vi "SFOAE-Compute Stim Spectra.vi"(0 "DataProc In":T1, 1 "MagSpect In":cluster{"Array":dbl[], "Array":dbl[]}[](array[cluster]), 11 "error in (no error)":errorcluster, 13 "Smoothing":cluster{"Length":i32, "Iterations":i32}={"Length"=1, "Iterations"=1}) -> (3 "MagSpect":cluster{"Array":dbl[], "Array":dbl[]}[](array[cluster]), 4 "DataProc Out":T1, 15 "error out":errorcluster)   [LabVIEW 2020]
uses:
  Typedefs/SFOAE-Data Processing.ctl
  <vilib>/Analysis/baseanly.llb/Mean (DBL).vi
  epl-vi-lib/Utility VIs/Math VIs/FFT x(t) to dB,Degrees (1D).vi
  epl-vi-lib/Utility VIs/Math VIs/Linear to dB (array).vi
  <vilib>/Analysis/NI_AALBase.lvlib
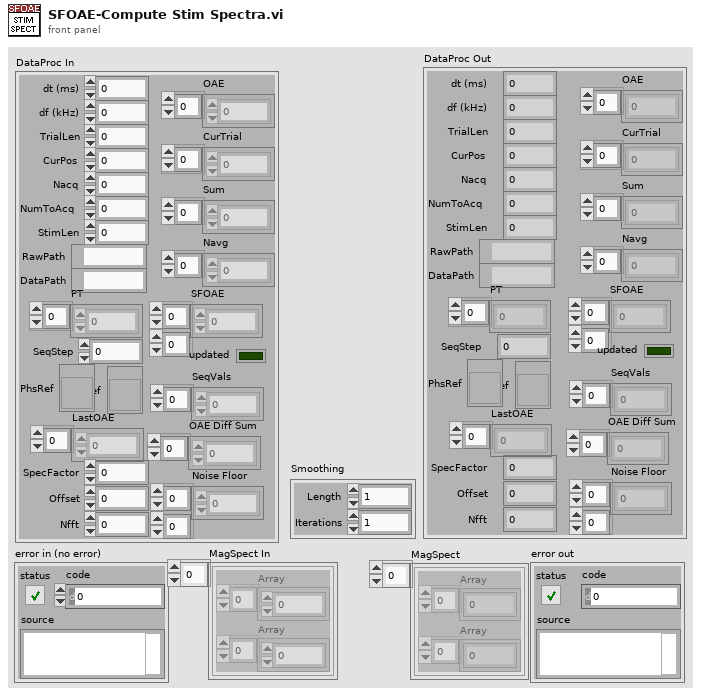
[diagram p1: front panel]
types:
  T1 = typedef "SFOAE-Data Processing.ctl" = cluster{"dt (ms)":dbl, "TrialLen":i32, "PT":cdb[], "CurPos":i32, "Sum":dbl[], "Navg":dbl[], "Nacq":i32, "RawPath":path, "DataPath":path, "NumToAcq":i32, "OAE":dbl[], "CurTrial":dbl[], "StimLen":i32, "SFOAE":cdb[][], "SeqStep":i32, "updated":bool, "SeqVals":dbl[], "df (kHz)":dbl, "MagRef":refnum<vi>, "LastOAE":dbl[], "OAE Diff Sum":dbl[], "Noise Floor":cdb[][], "SpecFactor":dbl, "Offset":i32, "Nfft":i32, "PhsRef":refnum<vi>}
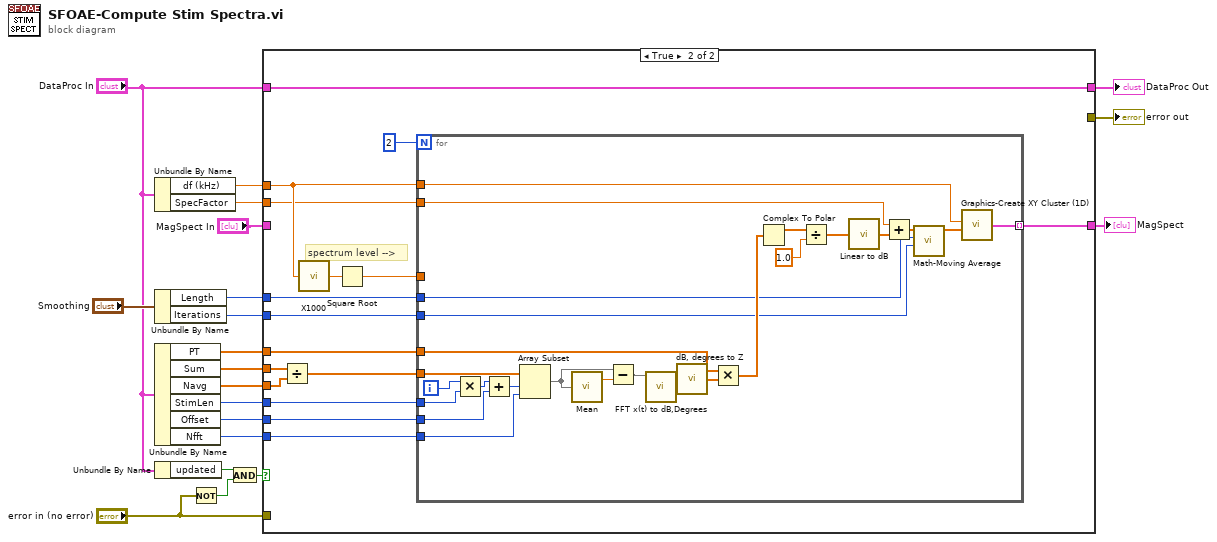
[diagram p0: block diagram]
diagram:
  n1 = Unbundle By Name("DataProc In") -> ("df (kHz)"=w13:dbl, "SpecFactor"=w8:dbl)
  n2 = Unbundle By Name("Smoothing") -> ("Length"=w11:i32, "Iterations"=w10:i32)
  n3 = Unbundle By Name("DataProc In") -> ("PT"=w6:cdb[], "Sum"=w14:dbl[], "Navg"=w7:dbl[], "StimLen"=w5:i32, "Offset"=w2:i32, "Nfft"=w1:i32)
  n4 = Unbundle By Name("DataProc In") -> ("updated"=w18:bool)
  n5 = Not(x="error in (no error)") -> (.not. x?=w17:bool)
  n6 = And(x=w18, y=w17) -> (x .and. y?=w15:bool)
  n7 = case shown="True" w15 {
    tunnel: "DataProc In" -> [w23 w33]
    tunnel: [w23 w33] -> w19
    tunnel: [w22 _] -> w20
    tunnel: "error in (no error)" -> [w22 _]
    tunnel: w14 -> [_ w32]
    tunnel: w13 -> [_ w37]
    tunnel: w11 -> [_ w38]
    tunnel: w10 -> [_ w39]
    tunnel: w8 -> [_ w34]
    tunnel: w7 -> [_ w31]
    tunnel: w6 -> [_ w29]
    tunnel: w5 -> [_ w28]
    tunnel: [w21 w27] -> w4
    tunnel: "MagSpect In" -> [w21 _]
    tunnel: w2 -> [_ w25]
    tunnel: w1 -> [_ w24]
    frame False {
    }
    frame True {
      # "spectrum level -->"
      n8 = Divide(x=w32, y=w31) -> (x/y=w30:dbl[])
      n9 = call "X1000.vi"("X"=w37) -> ("X/1000"=w35:dbl)
      n10 = Square Root(x=w35) -> (sqrt(x)=w36:dbl)
      n11 = for {
        N: 2 -> [_]
        tunnel: w39 -> [w58]
        tunnel: w38 -> [w57]
        tunnel: w37 -> [w55]
        tunnel: w36 -> [_]
        tunnel: w34 -> [w51]
        tunnel: w30 -> [w49]
        tunnel: w29 -> [w48]
        tunnel: w28 -> [w46]
        tunnel: [w44] -> w27 mode=indexing
        tunnel: w25 -> [w42]
        tunnel: w24 -> [w41]
        i -> [w45]
        n12 = Multiply(x=w45, y=w46) -> (x*y=w50:i32)
        n13 = Add(x=w50, y=w42) -> (x+y=w43:i32)
        n14 = Array Subset(array=w49, index=w43, length=w41) -> (w47:dbl[])
        n15 = call-poly <vilib>:"Mean.vi"("X"=w47) -> ("mean"=w54:dbl)  [unwired: 1 out]
        n16 = Subtract(x=w47, y=w54) -> (x-y=w53:dbl[])
        n17 = call-poly "FFT x(t) to dB,Degrees.vi"("X"=w53) -> ("+Freq Phase of FFT (degrees)"=w64:dbl[], "+Freq. Mag of FFT (dB rms)"=w65:dbl[])  [unwired: 8 in, 1 out]
        n18 = call "dB, degrees to Z.vi"("Magnitude (dB)"=w65, "Phase (degrees)"=w64) -> ("Z"=w63:cdb[])  [unwired: 5 in]
        n19 = Multiply(x=w48, y=w63) -> (x*y=w62:cdb[])
        n20 = Complex To Polar(r * e^(i*theta)=w62) -> (r=w61:dbl[])  [unwired: 1 out]
        n21 = Divide(x=w61, y=1.0) -> (x/y=w56:dbl[])
        n22 = call-poly "Linear to dB.vi"("linear"=w56) -> ("dB"=w59:dbl[])
        n23 = Add(x=w51, y=w59) -> (x+y=w52:dbl[])
        n24 = call "Math-Moving Average.vi"("Iterations"=w58, "Length"=w57, "Array in"=w52) -> ("Array out"=w60:dbl[])  [unwired: 8 in]
        n25 = call "Graphics-Create XY Cluster (1D).vi"("Array"=w60, "dx"=w55) -> ("XY cluster"=w44:cluster{"Array":dbl[], "Array":dbl[]})  [unwired: 2 in]
      }
    }
  }
  "error out" <- w20
  "DataProc Out" <- w19
  "MagSpect" <- w4
